vi "Driver Config Panel.vi"(8 "error in (no error)":errorcluster, 11 "Configuration In":string) -> (0 "error out":errorcluster, 2 "Serial Number":string, 3 "Configuration Out":string, 4 "LastCal":dbl, 6 "CalDue":dbl)   [LabVIEW 2011]
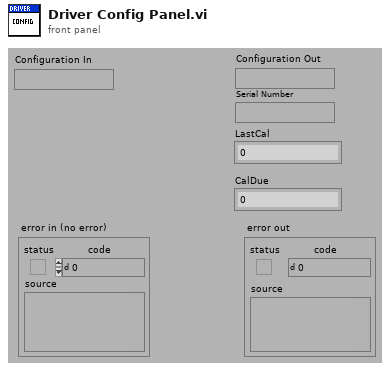
[diagram p1: front panel]
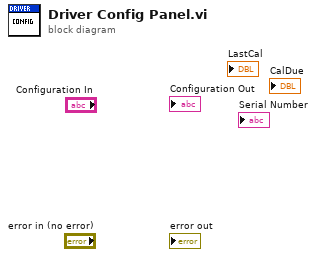
[diagram p0: block diagram]
diagram:
